vi "axis to drive.vi"(9 "X axis":i32, 10 "Y axis":i32, 11 "wej wagi":T1) -> (0 "wyj P":cluster{"y":dbl, "y":dbl, "y":dbl}, 3 "wyj L":cluster{"y":dbl, "y":dbl, "y":dbl})   [LabVIEW 2015]
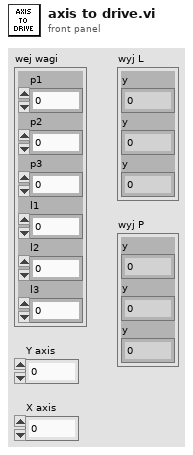
[diagram p1: front panel]
types:
  T1 = cluster{"p1":dbl, "p2":dbl, "p3":dbl, "l1":dbl, "l2":dbl, "l3":dbl}
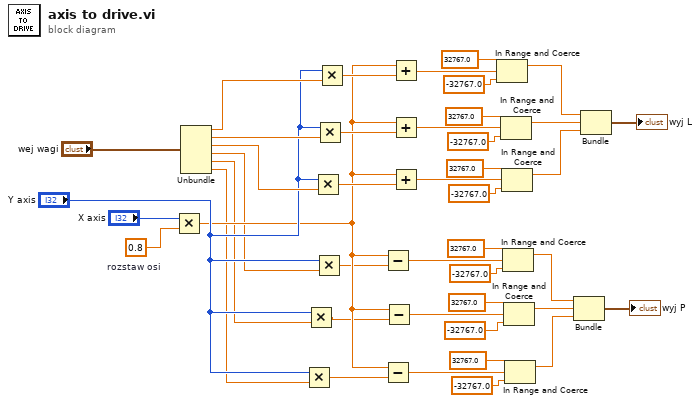
[diagram p0: block diagram]
diagram:
  w6 = 0.8  # rozstaw osi
  n1 = Multiply(x="X axis", y=w6) -> (x*y=w28:dbl)
  n2 = Unbundle("wej wagi") -> ("p1"=w30:dbl, "p2"=w31:dbl, "p3"=w32:dbl, "l1"=w19:dbl, "l2"=w20:dbl, "l3"=w21:dbl)
  n3 = Multiply(x="Y axis", y=w21) -> (x*y=w18:dbl)
  n4 = Multiply(x="Y axis", y=w20) -> (x*y=w17:dbl)
  n5 = Multiply(x="Y axis", y=w32) -> (x*y=w35:dbl)
  n6 = Multiply(x="Y axis", y=w19) -> (x*y=w16:dbl)
  n7 = Multiply(x="Y axis", y=w31) -> (x*y=w34:dbl)
  n8 = Multiply(x="Y axis", y=w30) -> (x*y=w33:dbl)
  n9 = Subtract(x=w28, y=w16) -> (x-y=w9:dbl)
  n10 = Subtract(x=w28, y=w18) -> (x-y=w15:dbl)
  n11 = Subtract(x=w28, y=w17) -> (x-y=w10:dbl)
  n12 = Add(x=w28, y=w33) -> (x+y=w27:dbl)
  n13 = Add(x=w28, y=w34) -> (x+y=w22:dbl)
  n14 = Add(x=w28, y=w35) -> (x+y=w8:dbl)
  n15 = In Range and Coerce(upper limit=32767.0 ("y"), x=w27, lower limit=-32767.0 ("y")) -> (coerced(x)=w36:dbl)  [unwired: 1 out]
  n16 = In Range and Coerce(upper limit=32767.0 ("y"), x=w22, lower limit=-32767.0 ("y")) -> (coerced(x)=w39:dbl)  [unwired: 1 out]
  n17 = In Range and Coerce(upper limit=32767.0 ("y"), x=w8, lower limit=-32767.0 ("y")) -> (coerced(x)=w37:dbl)  [unwired: 1 out]
  n18 = In Range and Coerce(upper limit=32767.0 ("y"), x=w9, lower limit=-32767.0 ("y")) -> (coerced(x)=w41:dbl)  [unwired: 1 out]
  n19 = In Range and Coerce(upper limit=32767.0 ("y"), x=w10, lower limit=-32767.0 ("y")) -> (coerced(x)=w42:dbl)  [unwired: 1 out]
  n20 = In Range and Coerce(upper limit=32767.0 ("y"), x=w15, lower limit=-32767.0 ("y")) -> (coerced(x)=w43:dbl)  [unwired: 1 out]
  n21 = Bundle("y"=w41, "y"=w42, "y"=w43) -> (→"wyj P":cluster{"y":dbl, "y":dbl, "y":dbl})  [unwired: 1 in]
  n22 = Bundle("y"=w36, "y"=w39, "y"=w37) -> (→"wyj L":cluster{"y":dbl, "y":dbl, "y":dbl})  [unwired: 1 in]
